vi "file name out DataAcq.vi"(1 "Data Acq":T1(ring)=enum."NML Data Acquisition-New.vi", 3 "command text in":string[](array[string])) -> (2 "file name out":string)   [LabVIEW 2025]
doc: "Author: Scott Hannahs <sth@magnet.fsu.edu>\n\nThis software is licensed for use under the “MIT License\"\nCopyright (c) 2025 Scott Hannahs, sth@sth@magnet.sthnet.net\n\nPermission is hereby granted, free of charge, to any person obtaining a copy of this software and associated documentation files (the \"Software\"), to deal in the Software without restriction, including without limitation the rights to use, copy, modify, merge, publish, distribute, sublicense, and/or sell copies of the Software, and to permit persons to whom the Software is furnished to do so, subject to the following conditions: The above copyright notice and this permission notice shall be included in all copies or substantial portions of the Software.\n\nTHE SOFTWARE IS PROVIDED \"AS IS\", WITHOUT WARRANTY OF ANY KIND, EXPRESS OR IMPLIED, INCLUDING BUT NOT LIMITED TO THE WARRANTIES OF MERCHANTABILITY, FITNESS FOR A PARTICULAR PURPOSE AND NONINFRINGEMENT. IN NO EVENT SHALL THE AUTHORS OR COPYRIGHT HOLDERS BE LIABLE FOR ANY CLAIM, DAMAGES OR OTHER LIABILITY, WHETHER IN AN ACTION OF CONTRACT, TORT OR OTHERWISE, ARISING FROM, OUT OF OR IN CONNECTION WITH THE SOFTWARE OR THE USE OR OTHER DEALINGS IN THE SOFTWARE."
panel:
  out "error out":errorcluster
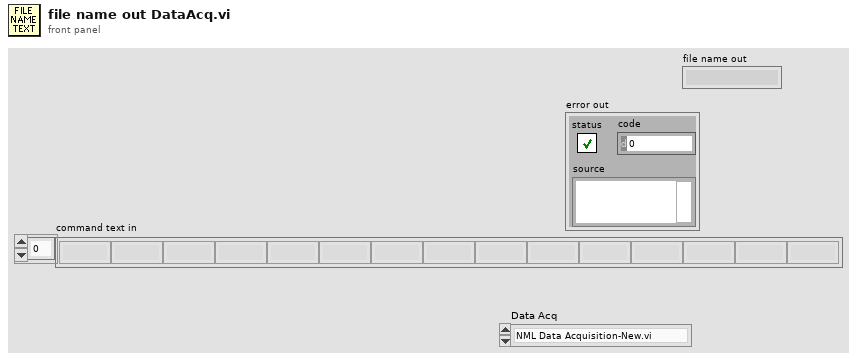
[diagram p1: front panel]
types:
  T1 = enum16{"NML Data Acquisition-old.vi", "NML Data Acquisition-New.vi"}
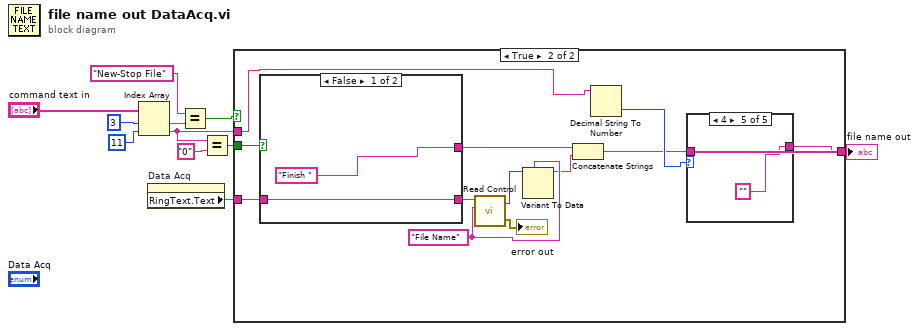
[diagram p0: block diagram]
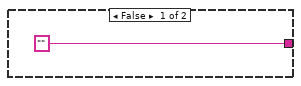
[diagram p2: hidden frame]
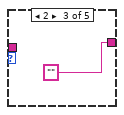
[diagram p5: hidden frame]
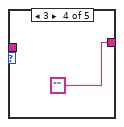
[diagram p6: hidden frame]
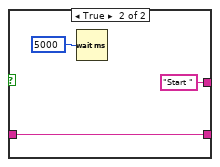
[diagram p7: hidden frame]
diagram:
  n1 = Index Array(array="command text in", index #1=3 ("index"), index #2=11 ("index")) -> (element #1=w9:string, element #2=w1:string)
  n2 = property on="Data Acq" class="Enum (strict)"() -> ("RingText.Text"=w2:string)  [unwired: 2 in, 2 out]
  n3 = Equal?(x="New-Stop File", y=w9) -> (x = y?=w10:bool)
  n4 = Equal?(x=w1, y="0") -> (x = y?=w4:bool)
  n5 = case shown="True" w10 {
    tunnel: ["" w14] -> w3
    tunnel: w4 -> [_ w24]
    tunnel: w2 -> [_ w23]
    tunnel: w1 -> [_ w16]
    frame False {
    }
    frame True {
      w21 = "File Name" ("VI Name")
      n6 = case shown="False" w24 {
        tunnel: w23 -> [w31 w34]
        tunnel: [w31 w34] -> w20
        tunnel: ["Finish " ("VI Name") "Start " ("VI Name")] -> w18
        frame False {
        }
        frame True {
          n7 = Wait (ms)(milliseconds to wait=u32 5000) -> ()  [unwired: 1 out]
        }
      }
      n8 = call "Read Control.vi"("VI Name"=w20, "Control Name"=w21) -> ("Value"=w22:variant, "error out"=→"error out":errorcluster)  [unwired: 3 in]
      n9 = Variant To Data(type=w21, Variant=w22) -> (data=w19:string)  [unwired: 1 in, 1 out]
      n10 = Concatenate Strings(w18, w19) -> (w13:string)
      n11 = Decimal String To Number(string=w16) -> (number=w15:i32)  [unwired: 2 in, 1 out]
      n12 = case shown="4" w15 {
        tunnel: [w25 w26 "" "" ""] -> w14
        tunnel: w13 -> [w25 w26 _ _ _]
        frame 0, Default {
        }
        frame 1 {
        }
        frame 2 {
        }
        frame 3 {
        }
        frame 4 {
        }
      }
    }
  }
  "file name out" <- w3
